vi "波形.vi"() -> ()   [LabVIEW 2015]
uses:
  <vilib>/measure/NI_MABase.lvlib
panel:
  out "波形长度":i32
  out "波形类型":string
  out "waveform out":waveform(dbl)
  out "size(s)":i32
  out "attributes":variant
  out "dt":dbl
  out "t0":timestamp
  out "Y":dbl[](array[numeric])
  out "Waveform Graph":waveform(dbl)(graph)
  in  "amplitude":dbl=1.0 format="%0.2p"
  in  "frequency":dbl=10.0 format="%0.2p"
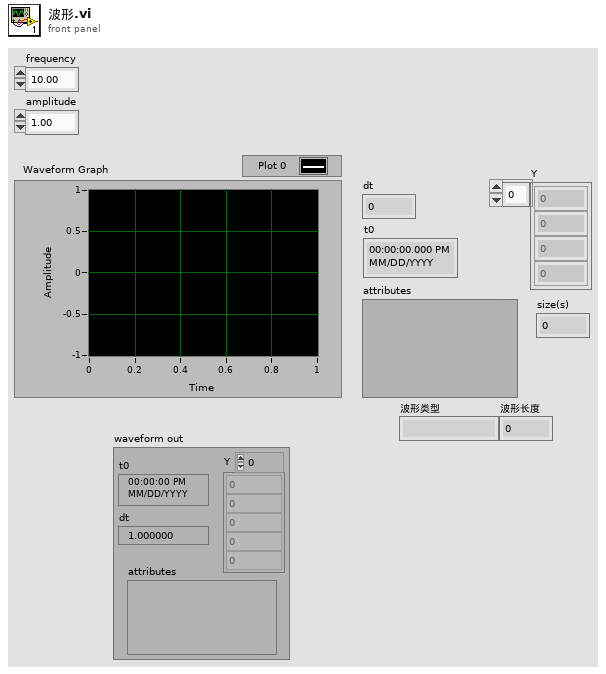
[diagram p1: front panel]
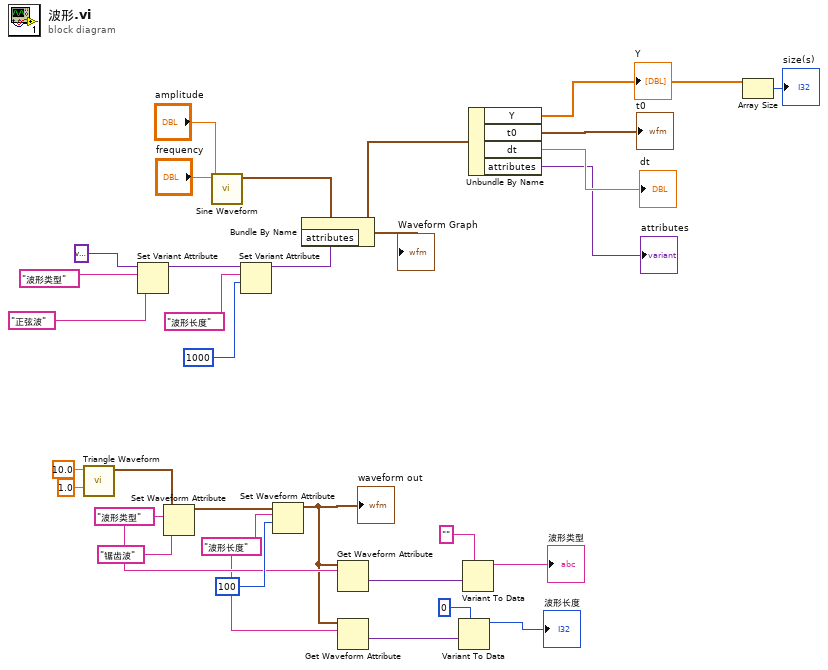
[diagram p0: block diagram]
diagram:
  w5 = "波形长度" ("name")
  w9 = "波形类型" ("name")
  n1 = call <vilib>:"Triangle Waveform.vi"("amplitude"=1.0, "frequency"=10.0) -> ("signal out"=w13:waveform(dbl))  [unwired: 8 in, 1 out]
  n2 = Set Variant Attribute(Variant=variant ("variant"), name="波形类型", value="正弦波" ("name")) -> (Variant out=w19:variant)  [unwired: 1 in, 2 out]
  n3 = Set Waveform Attribute(5:"锯齿波", 6:w9, 7:w13) -> (3:w11:waveform(dbl))  [unwired: 1 in, 2 out]
  n4 = call <vilib>:"Sine Waveform.vi"("amplitude"="amplitude", "frequency"="frequency") -> ("signal out"=w18:waveform(dbl))  [unwired: 8 in, 1 out]
  n5 = Set Variant Attribute(Variant=w19, name="波形长度", value=1000) -> (Variant out=w16:variant)  [unwired: 1 in, 2 out]
  n6 = Set Waveform Attribute(5:100, 6:w5, 7:w11) -> (3:w6:waveform(dbl))  [unwired: 1 in, 2 out]
  "waveform out" <- w6
  n7 = Bundle By Name(cluster=w18, "attributes"=w16) -> (w17:waveform(dbl))
  "Waveform Graph" <- w17
  n8 = Get Waveform Attribute(6:w9, 7:w6) -> (1:w8:variant)  [unwired: 2 in, 3 out]
  n9 = Get Waveform Attribute(6:w5, 7:w6) -> (1:w3:variant)  [unwired: 2 in, 3 out]
  n10 = Variant To Data(type=0, Variant=w3) -> (data=→"波形长度":i32)  [unwired: 1 in, 1 out]
  n11 = Variant To Data(type="", Variant=w8) -> (data=→"波形类型":string)  [unwired: 1 in, 1 out]
  n12 = Unbundle By Name(w17) -> ("Y"=w26:dbl[], "t0"=→"t0":timestamp, "dt"=→"dt":dbl, "attributes"=→"attributes":variant)
  "Y" <- w26
  n13 = Array Size(array=w26) -> (size(s)=→"size(s)":i32)
